vi "Force and Diameter Charts.vi"(8 "error in (no error)":errorcluster, 9 "gui notifier":refnum<notifier>, 10 "error queue":refnum<queue>, 11 "ia test notifier":refnum<notifier>) -> (0 "error out":errorcluster)   [LabVIEW 2020]
uses:
  Main GUI Loop/Handler.ctl
  Inflation Test/Result Handling/Inflation Test Numeric Results.ctl
panel:
  out "DIAMETER":cluster{dbl[], dbl[]}(graph) caption="diameter"
  out "force vs setpoint":cluster{dbl[], dbl[]}[](graph)
  # "FORCE VS. SETPOINT"
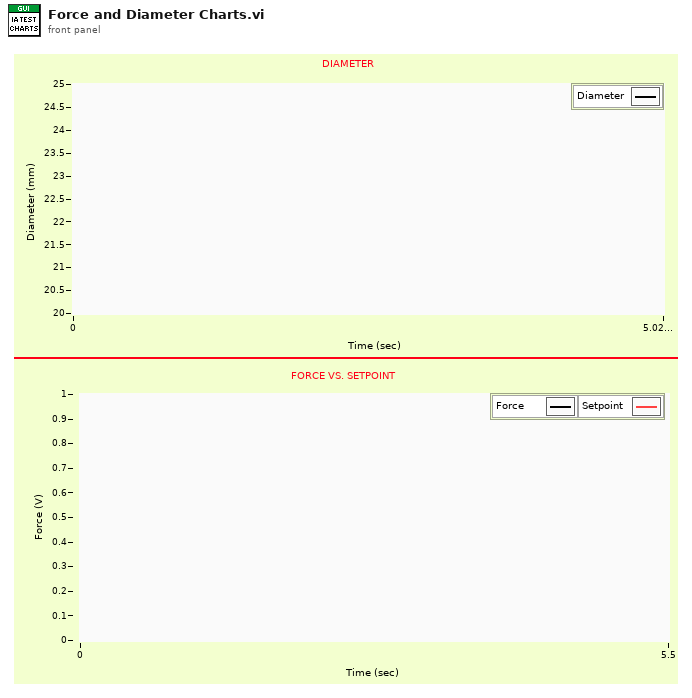
[diagram p1: front panel]
types:
  T1 = typedef "Inflation Test Numeric Results.ctl" = cluster{"diameter":dbl, "diam time":dbl, "force":dbl, "force time":dbl, "setpoint":dbl, "servo pw":dbl, "calibration log":dbl[][], "calibration results":dbl[][]}
  T2 = cluster{"appended array":dbl[], "appended array":dbl[]}
  T3 = cluster{"appended array":dbl[], "appended array":dbl[]}[]
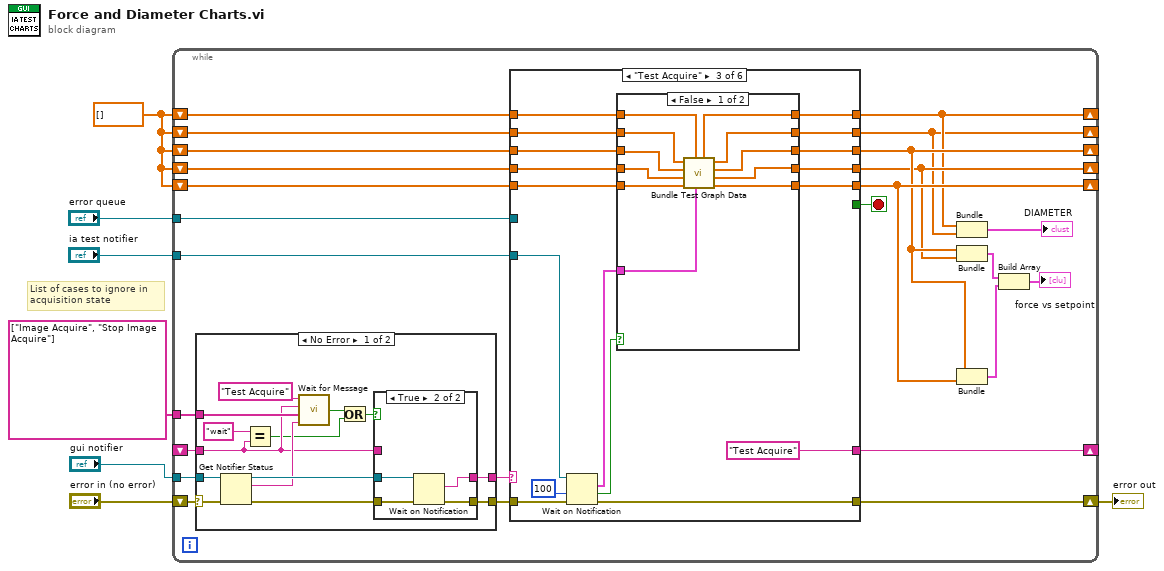
[diagram p0: block diagram]
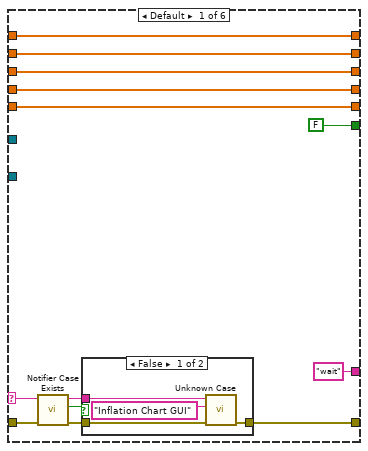
[diagram p2: hidden frame]
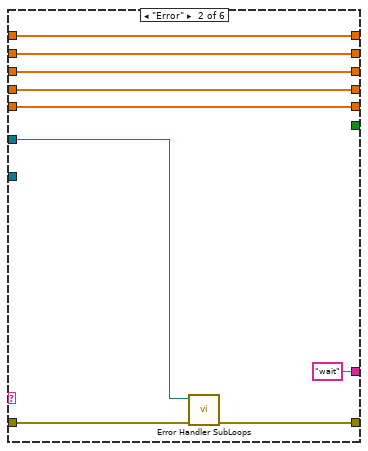
[diagram p4: hidden frame]
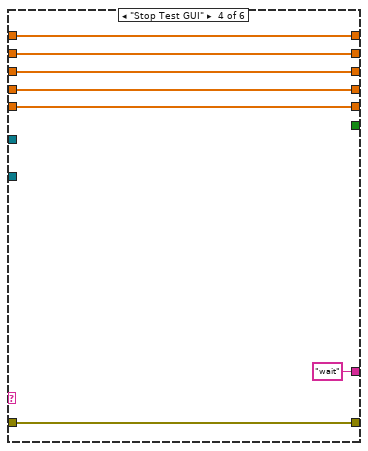
[diagram p6: hidden frame]
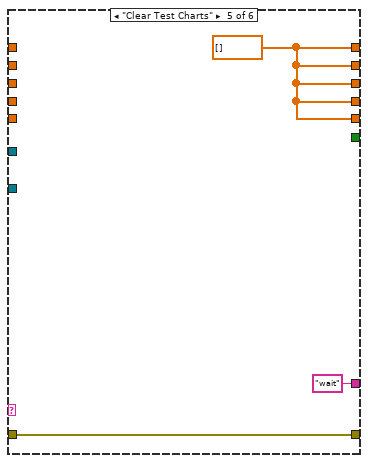
[diagram p7: hidden frame]
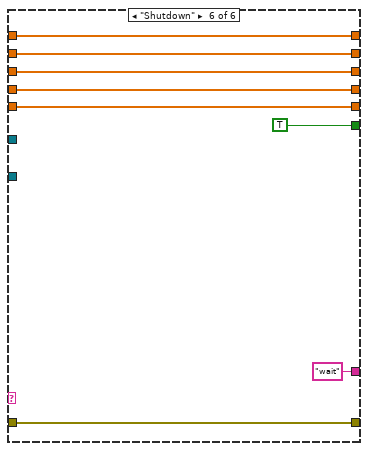
[diagram p8: hidden frame]
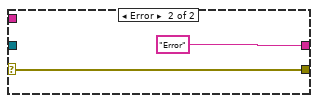
[diagram p10: hidden frame]
diagram:
  w2 = dbl[] [] ("appended array")
  # "List of cases to ignore in acquisition state"
  n1 = while {
    tunnel: "ia test notifier" -> [w31]
    tunnel: "gui notifier" -> [w30]
    shift-right: [w27] -> w5
    shift-left: "error in (no error)" -> [w29]
    tunnel: "error queue" -> [w25]
    shift-right: [w10] -> _
    shift-left: w2 -> [w24]
    shift-right: [w9] -> _
    shift-left: w2 -> [w23]
    shift-right: [w12] -> _
    shift-left: w2 -> [w22]
    shift-right: [w11] -> _
    shift-left: w2 -> [w21]
    shift-right: [w13] -> _
    shift-left: w2 -> [w20]
    shift-right: [w19] -> _
    shift-left: _ -> [w18]
    tunnel: string[] ["Image Acquire", "Stop Image Acquire"] ("x") -> [w8]
    stop <- w32 stop-if-true
    n2 = case shown="No Error" w29 {
      selector: w29 -> [w122 w132]
      tunnel: w30 -> [w120 _]
      tunnel: [w124 w132] -> w28
      tunnel: [w123 "Error" ("gui msg")] -> w26
      tunnel: w18 -> [w115 _]
      tunnel: w8 -> [w116 _]
      frame No Error {
        n3 = Get Notifier Status(notifier=w120, error in (no error)=w122) -> (notifier out=w119:refnum<notifier>, current notification=w117:string, error out=w121:errorcluster)  [unwired: 2 out]
        n4 = Equal?(x="wait", y=w115) -> (x = y?=w111:bool)
        n5 = call "Wait for Message.vi"("gui notification"=w117, "cases to ignore"=w116, "last state"=w115, "acquisition state name"="Test Acquire" ("t")) -> ("wait for notification?"=w113:bool)
        n6 = Or(x=w113, y=w111) -> (x .or. y?=w112:bool)
        n7 = case shown="True" w112 {
          tunnel: w119 -> [_ w130]
          tunnel: [w125 w129] -> w124
          tunnel: w121 -> [w125 w128]
          tunnel: [w126 w127] -> w123
          tunnel: w115 -> [w126 _]
          frame False {
          }
          frame True {
            n8 = Wait on Notification(notifier=w130, error in (no error)=w128) -> (notification=w127:string, error out=w129:errorcluster)  [unwired: 2 in, 2 out]
          }
        }
      }
      frame Error {
      }
    }
    n9 = case shown="\"Test Acquire\"" w26 {
      selector: w26 -> [w35 _ _ _ _ _]
      tunnel: [FALSE _ _ _ _ TRUE] -> w32
      tunnel: w31 -> [_ _ w76 _ _ _]
      tunnel: w28 -> [w37 w53 w75 w94 w101 w109]
      tunnel: [w44 w54 w74 w94 w101 w109] -> w27
      tunnel: w25 -> [_ w52 _ _ _ _]
      tunnel: w24 -> [w39 w55 w72 w95 _ w108]
      tunnel: w23 -> [w40 w56 w71 w96 _ w107]
      tunnel: w22 -> [w41 w57 w70 w97 _ w106]
      tunnel: w21 -> [w42 w58 w69 w98 _ w105]
      tunnel: w20 -> [w43 w59 w68 w99 _ w104]
      tunnel: [w39 w55 w67 w95 w102 w108] -> w10
      tunnel: [w40 w56 w66 w96 w102 w107] -> w9
      tunnel: [w41 w57 w65 w97 w102 w106] -> w12
      tunnel: [w42 w58 w64 w98 w102 w105] -> w11
      tunnel: [w43 w59 w63 w99 w102 w104] -> w13
      tunnel: ["wait" "wait" "Test Acquire" "wait" "wait" "wait"] -> w19
      frame Default {
        n10 = call "Notifier Case Exists.vi"("error in (no error)"=w37, "case in"=w35) -> ("error out"=w36:errorcluster, "defined case?"=w33:bool, "case out"=w34:string)  [unwired: 7 in]
        n11 = case shown="False" w33 {
          tunnel: [w49 w50] -> w44
          tunnel: w36 -> [w47 w50]
          tunnel: w34 -> [w46 _]
          frame False {
            n12 = call "Unknown Case.vi"("error in (no error)"=w47, "source"="Inflation Chart GUI", "case"=w46) -> ("error out"=w49:errorcluster)  [unwired: 8 in]
          }
          frame True {
          }
        }
      }
      frame "Error" {
        n13 = call "Error Handler SubLoops.vi"("error in"=w53, "main gui queue"=w52) -> ("error out"=w54:errorcluster)  [unwired: 9 in]
      }
      frame "Test Acquire" {
        n14 = Wait on Notification(notifier=w76, timeout in ms (-1)=100, error in (no error)=w75) -> (notification=w73:T1, timed out?=w61:bool, error out=w74:errorcluster)  [unwired: 1 in, 1 out]
        n15 = case shown="False" w61 {
          tunnel: w73 -> [w77 _]
          tunnel: w72 -> [w83 w92]
          tunnel: w71 -> [w84 w91]
          tunnel: w70 -> [w85 w90]
          tunnel: w69 -> [w86 w89]
          tunnel: w68 -> [w87 w88]
          tunnel: [w78 w92] -> w67
          tunnel: [w82 w91] -> w66
          tunnel: [w81 w90] -> w65
          tunnel: [w80 w89] -> w64
          tunnel: [w79 w88] -> w63
          frame False {
            n16 = call "Bundle Test Graph Data.vi"("ia test data"=w77, "diam time array in"=w83, "setpoint array in"=w87, "force array in"=w86, "force time array in"=w85, "diam array in"=w84) -> ("setpoint array out"=w79:dbl[], "force array out"=w80:dbl[], "force time array out"=w81:dbl[], "diam array out"=w82:dbl[], "diam time array out"=w78:dbl[])  [unwired: 1 in]
          }
          frame True {
            # "If no notifier is received from controller within 0.1sec, continue until a gui OR controller notification is received"
          }
        }
      }
      frame "Stop Test GUI" {
      }
      frame "Clear Test Charts" {
        w102 = dbl[] [] ("appended array")
      }
      frame "Shutdown" {
      }
    }
    n17 = Bundle("appended array"=w10, "appended array"=w9) -> (→"DIAMETER":T2)  [unwired: 1 in]
    n18 = Bundle("appended array"=w12, "appended array"=w11) -> (w15:T2)  [unwired: 1 in]
    n19 = Bundle("appended array"=w12, "appended array"=w13) -> (w14:T2)  [unwired: 1 in]
    n20 = Build Array(w15, w14) -> (→"force vs setpoint":T3)
  }
  "error out" <- w5
